vi "FPGA_refnum_to_session.vi"   [LabVIEW 2018]
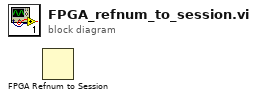
[diagram p0: block diagram]
diagram:
  n1 = FPGA Refnum to Session() -> ()  [unwired: 2 in, 2 out]
